vi "MFCcapability.vi"(10 "Ch Description":T3={"Ch Name"="", "Type"="", "Function"=enum."Analogue Input", "Ch State"=enum."On", "Calibration type"="", "A"=0.0, "B"=0.0, "C"=0.0, "D"=0.0, "Comments"="", "Address"={"Main"=0, "Ch."=0, "Sub"=0, "Port Name"=""}, "String"="", "Duty"=65535} {"Duty" format="%016b"; "D" format="%#_5g"; "C" format="%#_5g"; "B" format="%#_5g"; "A" format="%#_5g"}) -> (0 "MFCdescription":T1)   [LabVIEW 2016]
uses:
  ADAM Client/Sub VIs/ADAM Controls/Ch_description_ADAM.ctl
  ADAM Client/Sub VIs/ADAM Controls/Module_type_ADAM.ctl
  ADAM Client/Sub VIs/ADAM Controls/Function_ADAM.ctl
  ADAM Client/Sub VIs/ADAM Controls/Channel_State.ctl
  ADAM Client/Sub VIs/ADAM Controls/Calib_type_ADAM.ctl
  ADAM Client/Sub VIs/ADAM Controls/Address.ctl
  MFCdescription.ctl
  MFCcapability.ctl
panel:
  # "MFC calibration is Zero and Span:\nA is mass flow for 0% readout\nB is mass flow for 100% readout\n\nC is minimum recommended demand, %\nD is maximum recommended demand, %"
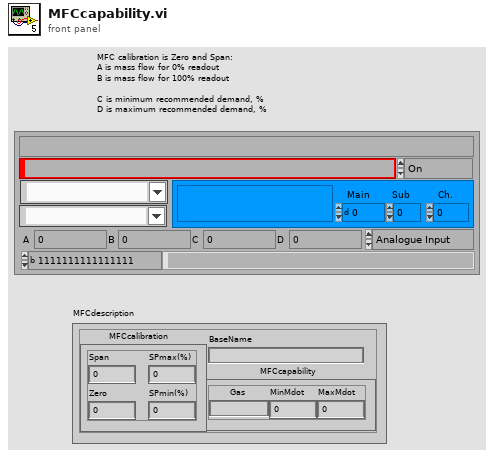
[diagram p1: front panel]
types:
  T1 = typedef "MFCdescription.ctl" = cluster{"BaseName":string, "MFCcalibration":cluster{"Span":dbl, "Zero":dbl, "SPmin(%)":dbl, "SPmax(%)":dbl}, "MFCcapability":T2}
  T2 = typedef "MFCcapability.ctl" = cluster{"Gas":string, "MinMdot":dbl, "MaxMdot":dbl}
  T3 = typedef "Ch_description_ADAM.ctl" = cluster{"Ch Name":string, "Type":T4, "Function":T5, "Ch State":T6, "Calibration type":T7, "A":dbl, "B":dbl, "C":dbl, "D":dbl, "Comments":string, "Address":T8, "String":string, "Duty":u16}
  T4 = typedef "Module_type_ADAM.ctl" = string
  T5 = typedef "Function_ADAM.ctl" = enum16{"Analogue Input", "Digital Input", "Event counter", "Event rate", "Analogue Output", "Digital Output", "Relay Output"}
  T6 = typedef "Channel_State.ctl" = enum16{"On", "Off", "Always On", "Always Off"}
  T7 = typedef "Calib_type_ADAM.ctl" = string
  T8 = typedef "Address.ctl" = cluster{"Main":i32, "Ch.":i32, "Sub":i32, "Port Name":string}
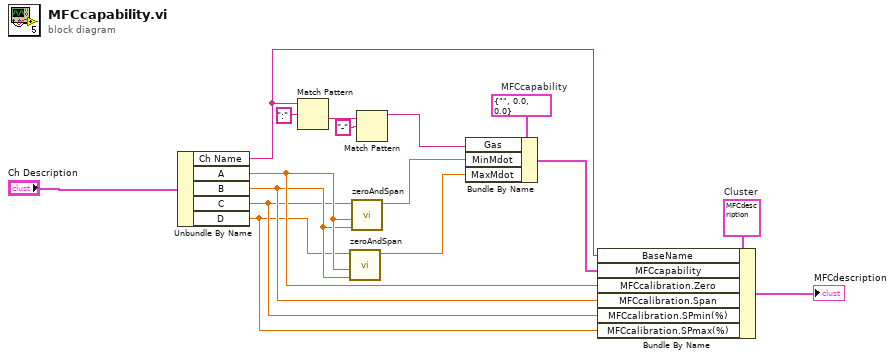
[diagram p0: block diagram]
diagram:
  w8 = T1 {"BaseName"="", "MFCcalibration"={"Span"=0.0, "Zero"=0.0, "SPmin(%)"=0.0, "SPmax(%)"=0.0}, "MFCcapability"={"Gas"="C2H6", "MinMdot"=1.0, "MaxMdot"=19.0}}  # Cluster
  w16 = T2 {"Gas"="", "MinMdot"=0.0, "MaxMdot"=0.0}  # MFCcapability
  n1 = Unbundle By Name("Ch Description") -> ("Ch Name"=w1:string, "A"=w7:dbl, "B"=w6:dbl, "C"=w5:dbl, "D"=w3:dbl)
  n2 = Match Pattern(string=w1, regular expression=":") -> (after substring=w12:string)  [unwired: 1 in, 3 out]
  n3 = call "zeroAndSpan.vi"("spanValue"=w6, "zeroValue"=w7, "MeasuredPercent"=w3) -> ("calibratedOutput"=w2:dbl)  [unwired: 6 in, 2 out]
  n4 = call "zeroAndSpan.vi"("spanValue"=w6, "zeroValue"=w7, "MeasuredPercent"=w5) -> ("calibratedOutput"=w4:dbl)  [unwired: 6 in, 2 out]
  n5 = Match Pattern(string=w12, regular expression="-") -> (before substring=w13:string)  [unwired: 1 in, 3 out]
  n6 = Bundle By Name(cluster=w16, "Gas"=w13, "MinMdot"=w4, "MaxMdot"=w2) -> (w9:T2)
  n7 = Bundle By Name(cluster=w8, "BaseName"=w1, "MFCcapability"=w9, "MFCcalibration.Zero"=w7, "MFCcalibration.Span"=w6, "MFCcalibration.SPmin(%)"=w5, "MFCcalibration.SPmax(%)"=w3) -> (→"MFCdescription":T1)
